vi "CTRE_Phoenix_MotorControl_SyncQuadratureWithPulseWidth.vi"(5 "Offset":i32, 6 "timeoutMs":u32, 7 "Cross Zero On Interval?":bool=TRUE, 8 "error in":errorcluster, 9 "Bookend 1":i32, 10 "Bookend 0":i32, 11 "PhoenixMotorControlDevRef":T1={"DeviceStatus"={"status"=FALSE, "code"=0, "source"=""}, "Type"=enum."PWM", "PWM"={"PWM Channel"=enum."Invalid", "DeadBand"={"Name"="", "maxPositivePwm"=0, "minPositivePwm"=0, "centerPwm"=0, "maxNegativePwm"=0, "minNegativePwm"=0, "angularRange"=0}}, "CAN"={"Device Number"=0, "SetOutput VI Ref"=variant(enum8{"Percent VBus", "Current", "Speed", "Position", "Voltage"} enum."Percent VBus"), "GetOutput VI Ref"=variant(refnum<k1> refnum), "Enable VI Ref"=variant(dbl 12.0), "Disable VI Ref"=variant(enum8{"Percent VBus", "Speed", "Position", "Slave", "Unchanged / Invalid", "Voltage Compensation", "Current", "Motion Profile"} enum."Percent VBus"), "Data"=variant}, "Invert"=FALSE, "DIO PWM"={"PWM \"Enable\" Channel"=enum."Invalid", "DIOChannel"=enum."Invalid", "PWM Rate"=0.0}}) -> (0 "Error Out":errorcluster, 3 "PhoenixMotorControlDevRef":T1={"DeviceStatus"={"status"=FALSE, "code"=0, "source"=""}, "Type"=enum."PWM", "PWM"={"PWM Channel"=enum."PWM 1", "DeadBand"={"Name"="", "maxPositivePwm"=0, "minPositivePwm"=0, "centerPwm"=0, "maxNegativePwm"=0, "minNegativePwm"=0, "angularRange"=0}}, "CAN"={"Device Number"=0, "SetOutput VI Ref"=variant(enum8{"Percent VBus", "Current", "Speed", "Position", "Voltage"} enum."Percent VBus"), "GetOutput VI Ref"=variant(refnum<k1> refnum), "Enable VI Ref"=variant(dbl 12.0), "Disable VI Ref"=variant(enum8{"Percent VBus", "Speed", "Position", "Slave", "Unchanged / Invalid", "Voltage Compensation", "Current", "Motion Profile"} enum."Percent VBus"), "Data"=variant}, "Invert"=FALSE, "DIO PWM"={"PWM \"Enable\" Channel"=enum."Invalid", "DIOChannel"=enum."Invalid", "PWM Rate"=0.0}})   [LabVIEW 2019]
uses:
  <vilib>/Rock Robotics/WPI/MotorControl/WPI_MotorControlDeviceRef.ctl
  <vilib>/Rock Robotics/WPI/MotorControl/WPI_MotorControlType.ctl
  <vilib>/Rock Robotics/SystemInterfaces/DIO/FPGA_DIOPWMChannel.ctl
  <vilib>/Rock Robotics/WPI/PWM/WPI_PWMDeadband.ctl
  <vilib>/Rock Robotics/SystemInterfaces/DIO/FPGA_DIOChannel.ctl
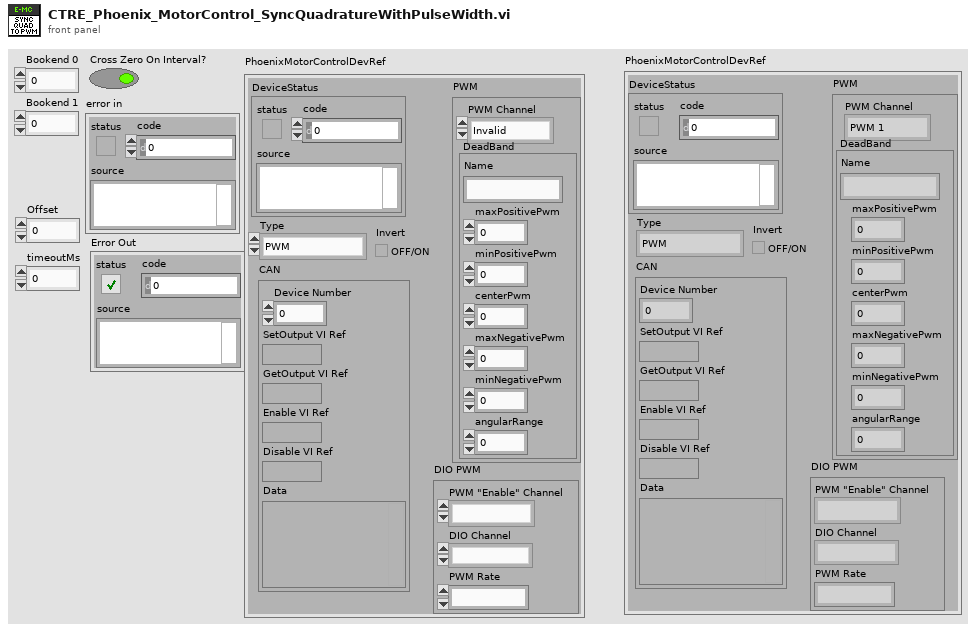
[diagram p1: front panel]
types:
  T1 = typedef "WPI_MotorControlDeviceRef.ctl" = cluster{"DeviceStatus":errorcluster, "Type":T2, "PWM":cluster{"PWM Channel":T3, "DeadBand":T4}, "CAN":cluster{"Device Number":u8, "SetOutput VI Ref":variant, "GetOutput VI Ref":variant, "Enable VI Ref":variant, "Disable VI Ref":variant, "Data":variant}, "Invert":bool, "DIO PWM":cluster{"PWM \"Enable\" Channel":T3, "DIOChannel":T5, "PWM Rate":dbl}}
  T2 = typedef "WPI_MotorControlType.ctl" = enum16{"PWM", "CAN", "DIO PWM"}
  T3 = typedef "FPGA_DIOPWMChannel.ctl" = enum8{"PWM 0", "PWM 1", "PWM 2", "PWM 3", "PWM 4", "PWM 5", "PWM 6", "PWM 7", "PWM 8", "PWM 9", "PWM MXP 0", "PWM MXP 1", "PWM MXP 2", "PWM MXP 3", "PWM MXP 4", "PWM MXP 5", "PWM MXP 6", "PWM MXP 7", "PWM MXP 8", "PWM MXP 9", "Invalid"}
  T4 = typedef "WPI_PWMDeadband.ctl" = cluster{"Name":string, "maxPositivePwm":i32, "minPositivePwm":i32, "centerPwm":i32, "maxNegativePwm":i32, "minNegativePwm":i32, "angularRange":u16}
  T5 = typedef "FPGA_DIOChannel.ctl" = enum8{"DIO 0", "DIO 1", "DIO 2", "DIO 3", "DIO 4", "DIO 5", "DIO 6", "DIO 7", "DIO 8", "DIO 9", "DIO MXP 0", "DIO MXP 1", "DIO MXP 2", "DIO MXP 3", "DIO MXP 4", "DIO MXP 5", "DIO MXP 6", "DIO MXP 7", "DIO MXP 8", "DIO MXP 9", "DIO MXP 10", "DIO MXP 11", "DIO MXP 12", "DIO MXP 13", "DIO MXP 14", "DIO MXP 15", "SPI Port CS1", "SPI Port CS2", "SPI Port CS3", "SPI Port MISO", "SPI Port MOSI", "Invalid"}
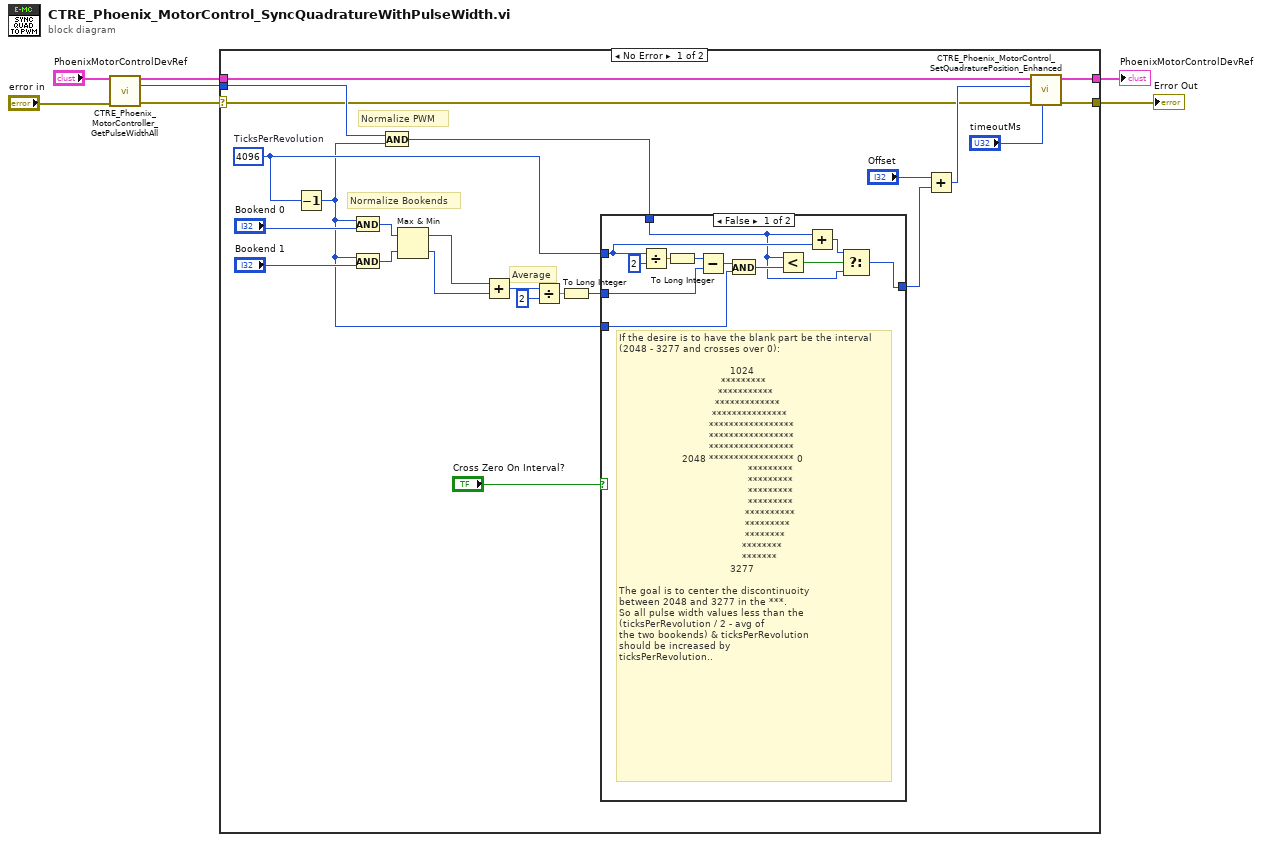
[diagram p0: block diagram]
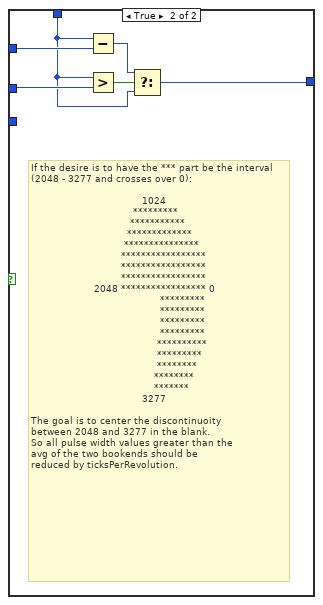
[diagram p2: hidden frame]
diagram:
  n1 = call <vilib>:"CTRE_Phoenix_MotorController_GetPulseWidthAll.vi"("PhoenixMotorControlDevRef"="PhoenixMotorControlDevRef", "error in"="error in") -> ("PhoenixMotorControlDevRef"=w5:T1, "Pulse Width Position"=w6:i32, "error out"=w2:errorcluster)  [unwired: 8 in, 3 out]
  n2 = case shown="No Error" w2 {
    selector: w2 -> [w8 w49]
    tunnel: w6 -> [w20 _]
    tunnel: w5 -> [w12 w50]
    tunnel: [w10 w50] -> w4
    tunnel: [w9 w49] -> w1
    frame No Error {
      w17 = 4096  # TicksPerRevolution
      # "Normalize PWM"
      # "Average"
      # "Normalize Bookends"
      n3 = Decrement(x=w17) -> (x-1=w16:i32)
      n4 = And(x=w16, y="Bookend 0") -> (x .and. y?=w28:i32)
      n5 = And(x=w16, y="Bookend 1") -> (x .and. y?=w27:i32)
      n6 = And(x=w20, y=w16) -> (x .and. y?=w18:i32)
      n7 = Max & Min(x=w28, y=w27) -> (max(x,y)=w25:i32, min(x,y)=w24:i32)
      n8 = Add(x=w25, y=w24) -> (x+y=w26:i32)
      n9 = Divide(x=w26, y=2) -> (x/y=w22:dbl)
      n10 = To Long Integer(number=w22) -> (32bit integer=w19:i32)
      n11 = case shown="False" "Cross Zero On Interval?" {
        tunnel: w19 -> [w36 w48]
        tunnel: w18 -> [w32 w44]
        tunnel: w17 -> [w33 w47]
        tunnel: [w31 w43] -> w15
        tunnel: w16 -> [w38 _]
        frame False {
          # "If the desire is to have the blank part be the interval \n(2048 - 3277 and crosses over 0): \n                                         \n                                     1024\n                                  *********    \n                                 ***********   \n                                *************  \n                               *************** \n                              *****************\n                              *****************\n                              *****************\n                     2048 ***************** 0\n                                           *********\n                                           *********\n                                           *********\n                                           *********\n                                          **********\n                                          ********* \n                                          ********  \n                                         ********   \n                                         *******\n                                     3277   \n             \nThe goal is to center the discontinuoity \nbetween 2048 and 3277 in the ***.\nSo all pulse width values less than the \n(ticksPerRevolution / 2 - avg of \nthe two bookends) & ticksPerRevolution \nshould be increased by \nticksPerRevolution.."
          n12 = Divide(x=w33, y=2) -> (x/y=w41:dbl)
          n13 = To Long Integer(number=w41) -> (32bit integer=w40:i32)
          n14 = Subtract(x=w40, y=w36) -> (x-y=w39:i32)
          n15 = And(x=w39, y=w38) -> (x .and. y?=w37:i32)
          n16 = Less?(x=w32, y=w37) -> (x < y?=w35:bool)
          n17 = Add(x=w32, y=w33) -> (x+y=w34:i32)
          n18 = Select(t=w34, s=w35, f=w32) -> (s? t:f=w31:i32)
        }
        frame True {
          # "If the desire is to have the *** part be the interval \n(2048 - 3277 and crosses over 0): \n                                         \n                                     1024\n                                  *********    \n                                 ***********   \n                                *************  \n                               *************** \n                              *****************\n                              *****************\n                              *****************\n                     2048 ***************** 0\n                                           *********\n                                           *********\n                                           *********\n                                           *********\n                                          **********\n                                          ********* \n                                          ********  \n                                         ********   \n                                         *******\n                                     3277   \n             \nThe goal is to center the discontinuoity \nbetween 2048 and 3277 in the blank.\nSo all pulse width values greater than the \navg of the two bookends should be \nreduced by ticksPerRevolution."
          n19 = Subtract(x=w44, y=w47) -> (x-y=w45:i32)
          n20 = Greater?(x=w44, y=w48) -> (0:w46:bool)
          n21 = Select(t=w45, s=w46, f=w44) -> (s? t:f=w43:i32)
        }
      }
      n22 = Add(x="Offset", y=w15) -> (x+y=w13:i32)
      n23 = call <vilib>:"CTRE_Phoenix_MotorControl_SetQuadraturePosition_Enhanced.vi"("timeoutMs"="timeoutMs", "error in (no error)"=w8, "New Position"=w13, "PhoenixMotorControlDevRef"=w12) -> ("error out"=w9:errorcluster, "PhoenixMotorControlDevRef"=w10:T1)  [unwired: 6 in]
    }
    frame Error {
    }
  }
  "PhoenixMotorControlDevRef" <- w4
  "Error Out" <- w1
